vi "Perform Evaluation.vi"(0 "Analyze BaseClass in":refnum<class "Analyze BaseClass.lvclass">, 5 "Image in":T1, 11 "error in (no error)":errorcluster) -> (4 "Analyze BaseClass out":refnum<class "Analyze BaseClass.lvclass">, 6 "Image out":T1, 8 "Result":refnum<class "Analyze Results Base.lvclass">, 15 "error out":errorcluster)   [LabVIEW 2014, in "Analyze.lvlib" / "Analyze BaseClass.lvlib" / "Analyze BaseClass.lvclass"]
uses:
  Analyze BaseClass.lvclass
  <vilib>/vision/Image Controls.llb/IMAQ Image.ctl
  Results and Overlays/Results Base/Analyze Results Base.lvclass
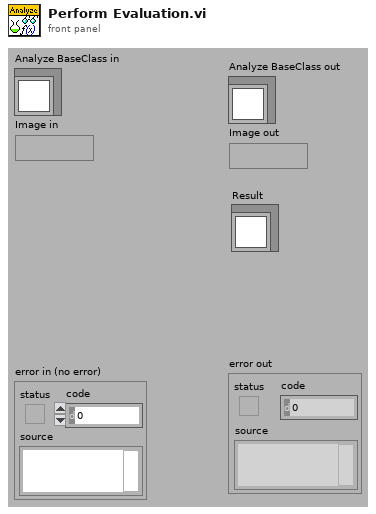
[diagram p1: front panel]
types:
  T1 = typedef "IMAQ Image.ctl" = refnum<image>
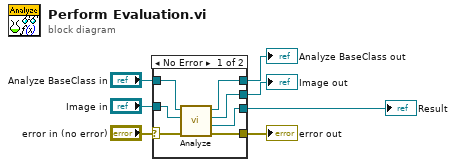
[diagram p0: block diagram]
diagram:
  n1 = case shown="No Error" "error in (no error)" {
    selector: "error in (no error)" -> [w12 w17]
    tunnel: [w11 w17] -> w6
    tunnel: [w13 w16] -> w4
    tunnel: "Analyze BaseClass in" -> [w14 w16]
    tunnel: "Image in" -> [w10 w15]
    tunnel: [w9 w15] -> w2
    tunnel: [w8 _] -> w1
    frame No Error {
      n2 = call-dynamic "Analyze.vi"("error in (no error)"=w12, "Image in"=w10, "Analyze BaseClass in"=w14) -> ("error out"=w11:errorcluster, "Result"=w8:refnum<class "Analyze Results Base.lvclass">, "Image out"=w9:T1, "Analyze BaseClass out"=w13:refnum<class "Analyze BaseClass.lvclass">)  [unwired: 5 in]
    }
    frame Error {
    }
  }
  "error out" <- w6
  "Analyze BaseClass out" <- w4
  "Image out" <- w2
  "Result" <- w1
